vi "Multiple_JSON_READ.vi"(2 "Json File Path":path, 7 "ERD Data Out":cluster{"ERD Number":u16, "Data":string}[](array[cluster]) {"ERD Number" format="%.0x"}, 11 "error in":errorcluster) -> (6 "Multiple JSON Data":cluster{"ERD Number":u16, "Data":string}[](array[cluster]), 15 "error out":errorcluster)   [LabVIEW 2021]
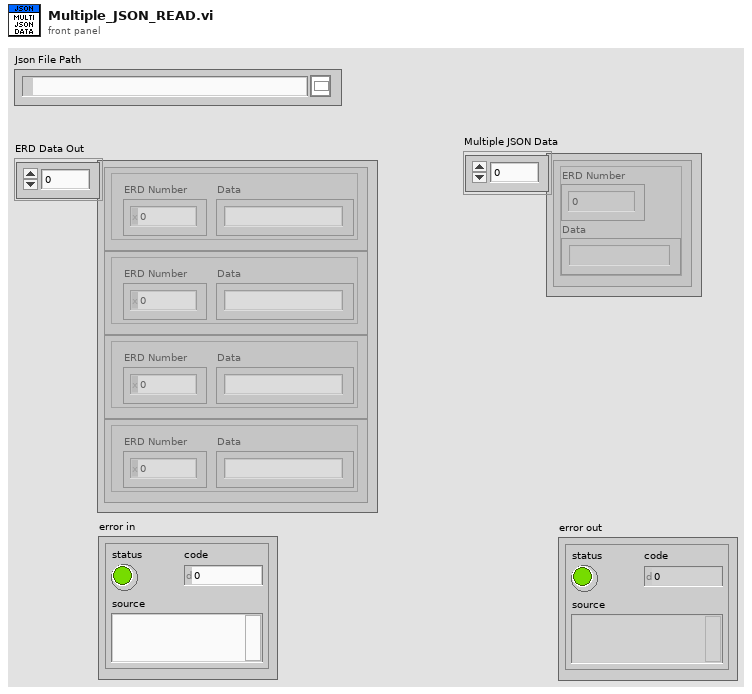
[diagram p1: front panel]
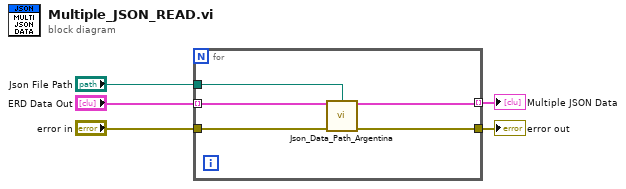
[diagram p0: block diagram]
diagram:
  n1 = for {
    tunnel: "ERD Data Out" -> [w10] mode=indexing
    tunnel: "error in" -> [w9]
    tunnel: "Json File Path" -> [w8]
    tunnel: [w7] -> w2 mode=indexing
    tunnel: [w6] -> w1
    n2 = call "Json_Data_Path_Argentina.vi"("ERD Cluster"=w10, "Json File Path"=w8, "error in"=w9) -> ("ERD JSON"=w7:cluster{"ERD Number":u16, "Data":string}, "error out"=w6:errorcluster)  [unwired: 11 in]
  }
  "Multiple JSON Data" <- w2
  "error out" <- w1
